vi "Drive Controller.vi"(8 "error in":errorcluster) -> ()   [LabVIEW 2017]
doc: "This VI executes continuously carrying out the current operation and responding to updates or new operation requests. It will often contain the timing or control code that is difficult to place directly in TeleOp. This VI generally opens all sensors and motors and isolates the rest of the robot code from knowing implementation details of how the operations are carried out."
uses:
  <vilib>/Rock Robotics/WPI/Framework/Completion Status.ctl
  Drive Setpoints.ctl
  Drive Operations.ctl
  Shared/RobotNeededPathData.ctl
  <vilib>/Rock Robotics/WPI/SafetyOutput/WPI_SafetyOutputConfigMenu.ctl
  <vilib>/Rock Robotics/SystemInterfaces/DIO/FPGA_DIOPWMChannel.ctl
  <vilib>/Rock Robotics/SystemInterfaces/DIO/FPGA_DIOChannel.ctl
  <vilib>/Rock Robotics/WPI/DriverStation/WPI_DriverStationRobotMode2.ctl
  <vilib>/Rock Robotics/WPI/ThirdParty/Sensors/navX/_TypeDefs/FRIC_navX_DeviceNumbersTypeDef.ctl
  <vilib>/Rock Robotics/WPI/RobotDrive/WPI_RobotDriveOpen4MotorWithSPARK.vi
  <vilib>/Rock Robotics/WPI/Counter/WPI_CounterDigitalInputToDigitalSource.vi
  <vilib>/Rock Robotics/WPI/RobotDrive/WPI_RobotDriveOpen2MotorWithSPARK.vi
  <vilib>/Rock Robotics/Network Tables/NT Write Number.vi
  Framework/Robot Global Data.vi
  Drive Published Globals.vi
  <vilib>/addons/control/pid/pid.llb/PID (DBL).vi
  <vilib>/addons/control/pid/NI_PID_pid.lvlib
  Configuration/Constants.vi
panel:
  in  "Integral Range":dbl=15.0
  out "PID Tuining":cluster{dbl, dbl}(graph)={170.0, 167.02}
  in  "Points":cluster{"X":dbl, "Y":dbl}[](array[cluster])=[{"X"=0.0, "Y"=0.0}, {"X"=0.01, "Y"=0.0}, {"X"=0.011, "Y"=0.17}, {"X"=1.0, "Y"=1.0}]
  in  "PID gains":T1={"proportional gain (Kc)"=0.01, "integral time (Ti, min)"=0.007, "derivative time (Td, min)"=0.0015} {"derivative time (Td, min)" format="%#_9g"}
  in  "Gains":T2={"FFV"=0.0059, "FFA"=0.0019, "Vel PID"={"P"=0.01, "I"=0.0, "D"=0.0}}
  in  "Interactive Values":T3={"Operation"=enum."Turn to Angle", "Left Speed"=-0.27, "Right Speed"=0.27, "Duration"=2.0, "Speed"=0.0, "Start Angle"=0.0, "Target Angle"=180.0, "Distance (inch)"=0.0, "Start Point (inch)"=0.0, "RobotNeededPathData"={"Path"=[], "MaxVel"=0.0, "MaxAccel"=-1.0, "Backwards?"=FALSE, "PointSpacing"=0.0, "LookaheadDist"=0.0, "Speed/Curve"=1.8, "SlowDistanceAtEnd"=12.0, "SlowSpeed"=15.0, "MaxDeAccel"=0.0}, "Start Point 2"=0.0} {"RobotNeededPathData"."SlowSpeed" format="%#_13g"; "RobotNeededPathData"."SlowDistanceAtEnd" format="%#_13g"; "RobotNeededPathData"."Speed/Curve" format="%#_13g"}
  in  "Buttons":cluster{"Execute Cmd":bool, "Abort Cmd":bool}
  out "Command Timing":cluster{"Start Time (ms)":u32, "Iterations":i32}={"Start Time (ms)"=372507, "Iterations"=0}
  out "Status":T6
  out "Setpoints":T7(graph)
  out "Current\nCmd":string="Started at  14:51:47.884\nDefault: Reserve,  L 0.0, R 0.0, D 0.000000"
  # "Tip: The graph shows the motor setpoints. It may also be helpful to observe inputs and sensor values.\nYou may also want to display tuning or debugging controls."
  # ".0088"
  # ".0017"
  # ".02"
  # "Interactive Command: You may fill in the settings for a command\nand schedule it with the Execute button. You can observe and abort\nany command while fine tuning the code for the controller."
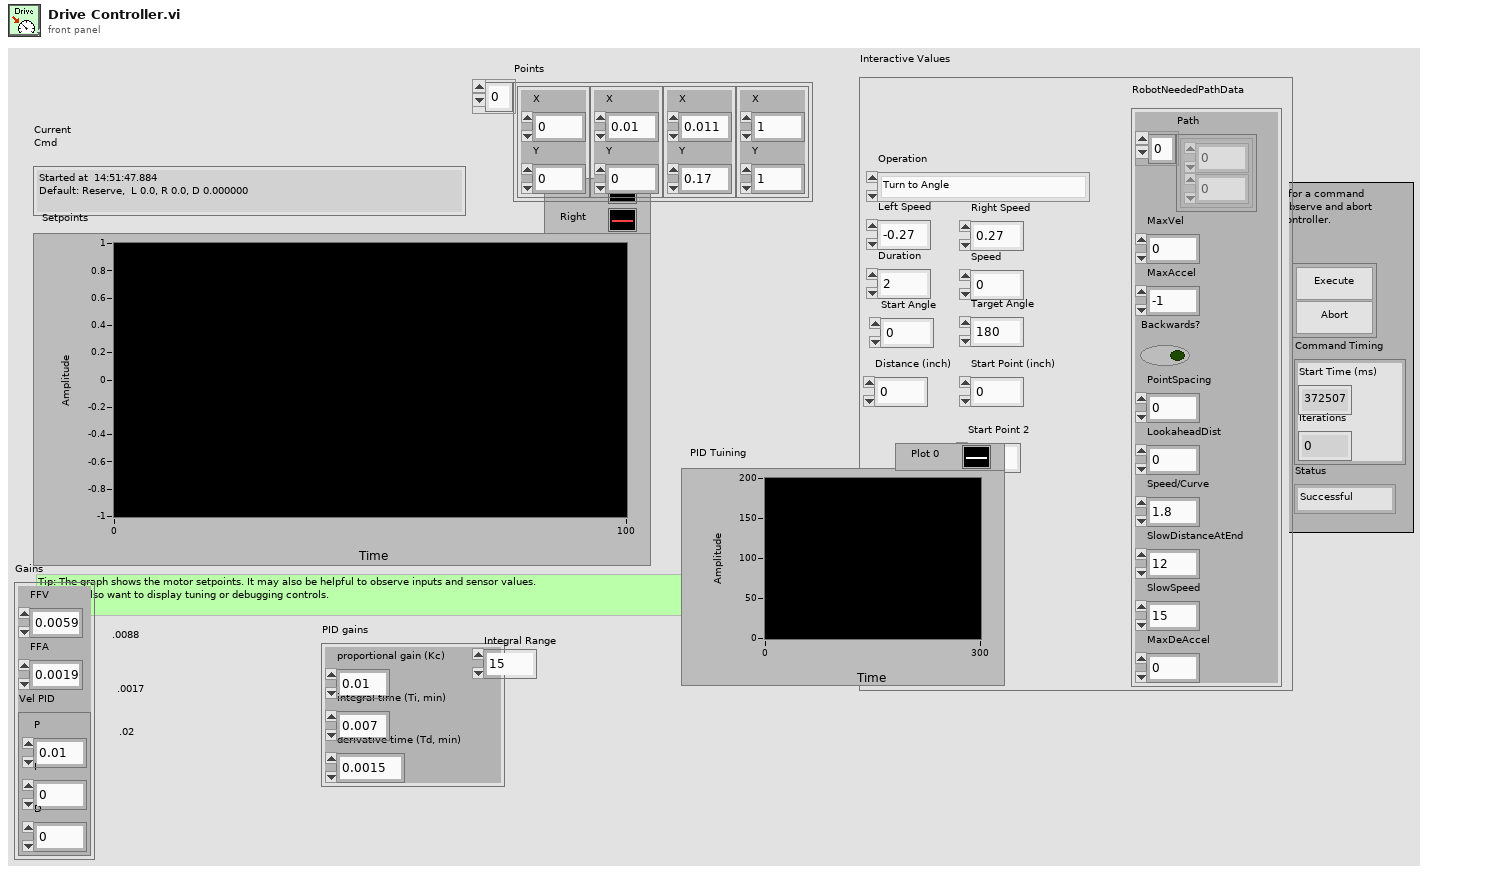
[diagram p1: front panel]
types:
  T1 = cluster{"proportional gain (Kc)":dbl, "integral time (Ti, min)":dbl, "derivative time (Td, min)":dbl}
  T2 = cluster{"FFV":dbl, "FFA":dbl, "Vel PID":cluster{"P":dbl, "I":dbl, "D":dbl}}
  T3 = typedef "Drive Setpoints.ctl" = cluster{"Operation":T4, "Left Speed":dbl, "Right Speed":dbl, "Duration":dbl, "Speed":dbl, "Start Angle":dbl, "Target Angle":dbl, "Distance (inch)":dbl, "Start Point (inch)":dbl, "RobotNeededPathData":T5, "Start Point 2":dbl}
  T4 = typedef "Drive Operations.ctl" = enum16{"Reserve", "Read Current", "Immediate", "Drive for Time", "Drive for Distance", "Turn to Angle", "Arc Turn", "Drive Path", "Drive To Cube"}
  T5 = typedef "RobotNeededPathData.ctl" = cluster{"Path":cluster{dbl, dbl}[], "MaxVel":dbl, "MaxAccel":dbl, "Backwards?":bool, "PointSpacing":dbl, "LookaheadDist":dbl, "Speed/Curve":dbl, "SlowDistanceAtEnd":dbl, "SlowSpeed":dbl, "MaxDeAccel":dbl}
  T6 = typedef "Completion Status.ctl" = enum16{"Successful", "Aborted", "Incomplete"}
  T7 = cluster{"Left Setpoint":dbl, "Right Setpoint":dbl}
  T8 = typedef "FPGA_DIOChannel.ctl" = enum8{"DIO 0", "DIO 1", "DIO 2", "DIO 3", "DIO 4", "DIO 5", "DIO 6", "DIO 7", "DIO 8", "DIO 9", "DIO MXP 0", "DIO MXP 1", "DIO MXP 2", "DIO MXP 3", "DIO MXP 4", "DIO MXP 5", "DIO MXP 6", "DIO MXP 7", "DIO MXP 8", "DIO MXP 9", "DIO MXP 10", "DIO MXP 11", "DIO MXP 12", "DIO MXP 13", "DIO MXP 14", "DIO MXP 15", "SPI Port CS1", "SPI Port CS2", "SPI Port CS3", "SPI Port MISO", "SPI Port MOSI", "Invalid"}
  T9 = typedef "FPGA_DIOPWMChannel.ctl" = enum8{"PWM 0", "PWM 1", "PWM 2", "PWM 3", "PWM 4", "PWM 5", "PWM 6", "PWM 7", "PWM 8", "PWM 9", "PWM MXP 0", "PWM MXP 1", "PWM MXP 2", "PWM MXP 3", "PWM MXP 4", "PWM MXP 5", "PWM MXP 6", "PWM MXP 7", "PWM MXP 8", "PWM MXP 9", "Invalid"}
  T10 = typedef "WPI_SafetyOutputConfigMenu.ctl" = enum16{"Enable", "Disable"}
  T11 = typedef "WPI_DigitalInputDevRef.ctl" = cluster{"DevStatus":errorcluster, "DIO Channel":T8}
  T12 = typedef "FPGA_CounterEncoderSourceConvertionLVSourceType.ctl" = cluster{"DevStatus":errorcluster, "AnalogTriggerMode?":bool, "DigitalMode":cluster{"DIO Channel":T13}, "AnalogTriggerMode":cluster{"AnalogTriggerIndex":T14, "OutputType":T15}}
  T13 = typedef "FPGA_DIODigitalSourceChannel.ctl" = enum8{"DIO 0", "DIO 1", "DIO 2", "DIO 3", "DIO 4", "DIO 5", "DIO 6", "DIO 7", "DIO 8", "DIO 9", "DIO MXP 0", "DIO MXP 1", "DIO MXP 2", "DIO MXP 3", "DIO MXP 4", "DIO MXP 5", "DIO MXP 6", "DIO MXP 7", "DIO MXP 8", "DIO MXP 9", "DIO MXP 10", "DIO MXP 11", "DIO MXP 12", "DIO MXP 13", "DIO MXP 14", "DIO MXP 15", "Disabled"}
  T14 = typedef "FPGA_AnalogTriggerIndex.ctl" = enum8{"Trig 0", "Trig 1", "Trig 2", "Trig 3", "Trig 4", "Trig 5", "Trig 6", "Trig 7", "Invalid"}
  T15 = typedef "FPGA_AnalogTriggerOutType.ctl" = enum16{"InWindow", "TriggerState", "Rising", "Falling"}
  T16 = typedef "WPI_RobotDriveDevRef.ctl" = cluster{"DevStatus":errorcluster, "Motors[]":T17[], "Square Inputs":bool, "Max Output":dbl}
  T17 = typedef "WPI_MotorControlDeviceRef.ctl" = cluster{"DeviceStatus":errorcluster, "Type":T18, "PWM":cluster{"PWM Channel":T9, "DeadBand":T19}, "CAN":cluster{"Device Number":u8, "SetOutput VI Ref":variant, "GetOutput VI Ref":variant, "Enable VI Ref":variant, "Disable VI Ref":variant, "Data":variant}, "Invert":bool, "DIO PWM":cluster{"PWM \"Enable\" Channel":T9, "DIOChannel":T8, "PWM Rate":dbl}}
  T18 = typedef "WPI_MotorControlType.ctl" = enum16{"PWM", "CAN", "DIO PWM"}
  T19 = typedef "WPI_PWMDeadband.ctl" = cluster{"Name":string, "maxPositivePwm":i32, "minPositivePwm":i32, "centerPwm":i32, "maxNegativePwm":i32, "minNegativePwm":i32, "angularRange":u16}
  T20 = typedef "WPI_EncoderDevRef.ctl" = cluster{"DevStatus":errorcluster, "EncoderIndex":T21, "CounterIndex":T22, "DistancePerCount":dbl, "Decoding Type":T23}
  T21 = typedef "FPGA_EncoderIdx.ctl" = enum8{"Enc 0", "Enc 1", "Enc 2", "Enc 3", "Enc 4", "Enc 5", "Enc 6", "Enc 7", "Invalid"}
  T22 = typedef "FPGA_CounterCtrSystemIndex.ctl" = enum8{"Ctr 0", "Ctr 1", "Ctr 2", "Ctr 3", "Ctr 4", "Ctr 5", "Ctr 6", "Ctr 7", "Invalid"}
  T23 = typedef "WPI_EncoderType.ctl" = enum16{"1x", "2x", "4x"}
  T24 = typedef "Command Status Info.ctl" = cluster{"Name":string, "Status":T6, "notifier out":T25}
  T25 = typedef "Completion Notifier.ctl" = refnum<notifier>
  T26 = cluster{"SubSystem Data":T3, cluster{"Start Time (ms)":u32, "Iterations":i32}, cluster{"Command Info":T24, "Description":string, "Default Command":T3, "queue out":refnum<queue>, "Subsystem Name":string}}
  T27 = typedef "WPI_DriverStationRobotMode2.ctl" = enum16{"Autonomous Disabled", "Autonomous Enabled", "Teleop Disabled", "Teleop Enabled", "Disconnected", "Finish", "Test Disabled", "Test Enabled", "Emergency Stopped"}
  T28 = cluster{"Yaw":dbl, "Roll":dbl, "Pitch":dbl, "Heading":dbl, "Fused Heading":dbl}
  T29 = typedef "FRIC_navX_DeviceNumbersTypeDef.ctl" = enum16{"Dev0", "Dev1", "Dev2", "Dev3"}
  T30 = cluster{"dx/dt":dbl, "dx/dt":dbl, "Yaw":dbl, cluster{dbl, dbl}}
  T31 = cluster{"LeftDistance":dbl, "RightDistance":dbl, "LeftVelocity":dbl, "RightVelocity":dbl, "Angle":dbl, "Location":cluster{dbl, dbl}}
  T32 = cluster{"SubSystem Data":T3, cluster{"Start Time (ms)":u32, "Iterations":i32}, "Default Command Arguments":cluster{"Command Info":T24, "Description":string, "Default Command":T3, "queue out":refnum<queue>, "Subsystem Name":string}}
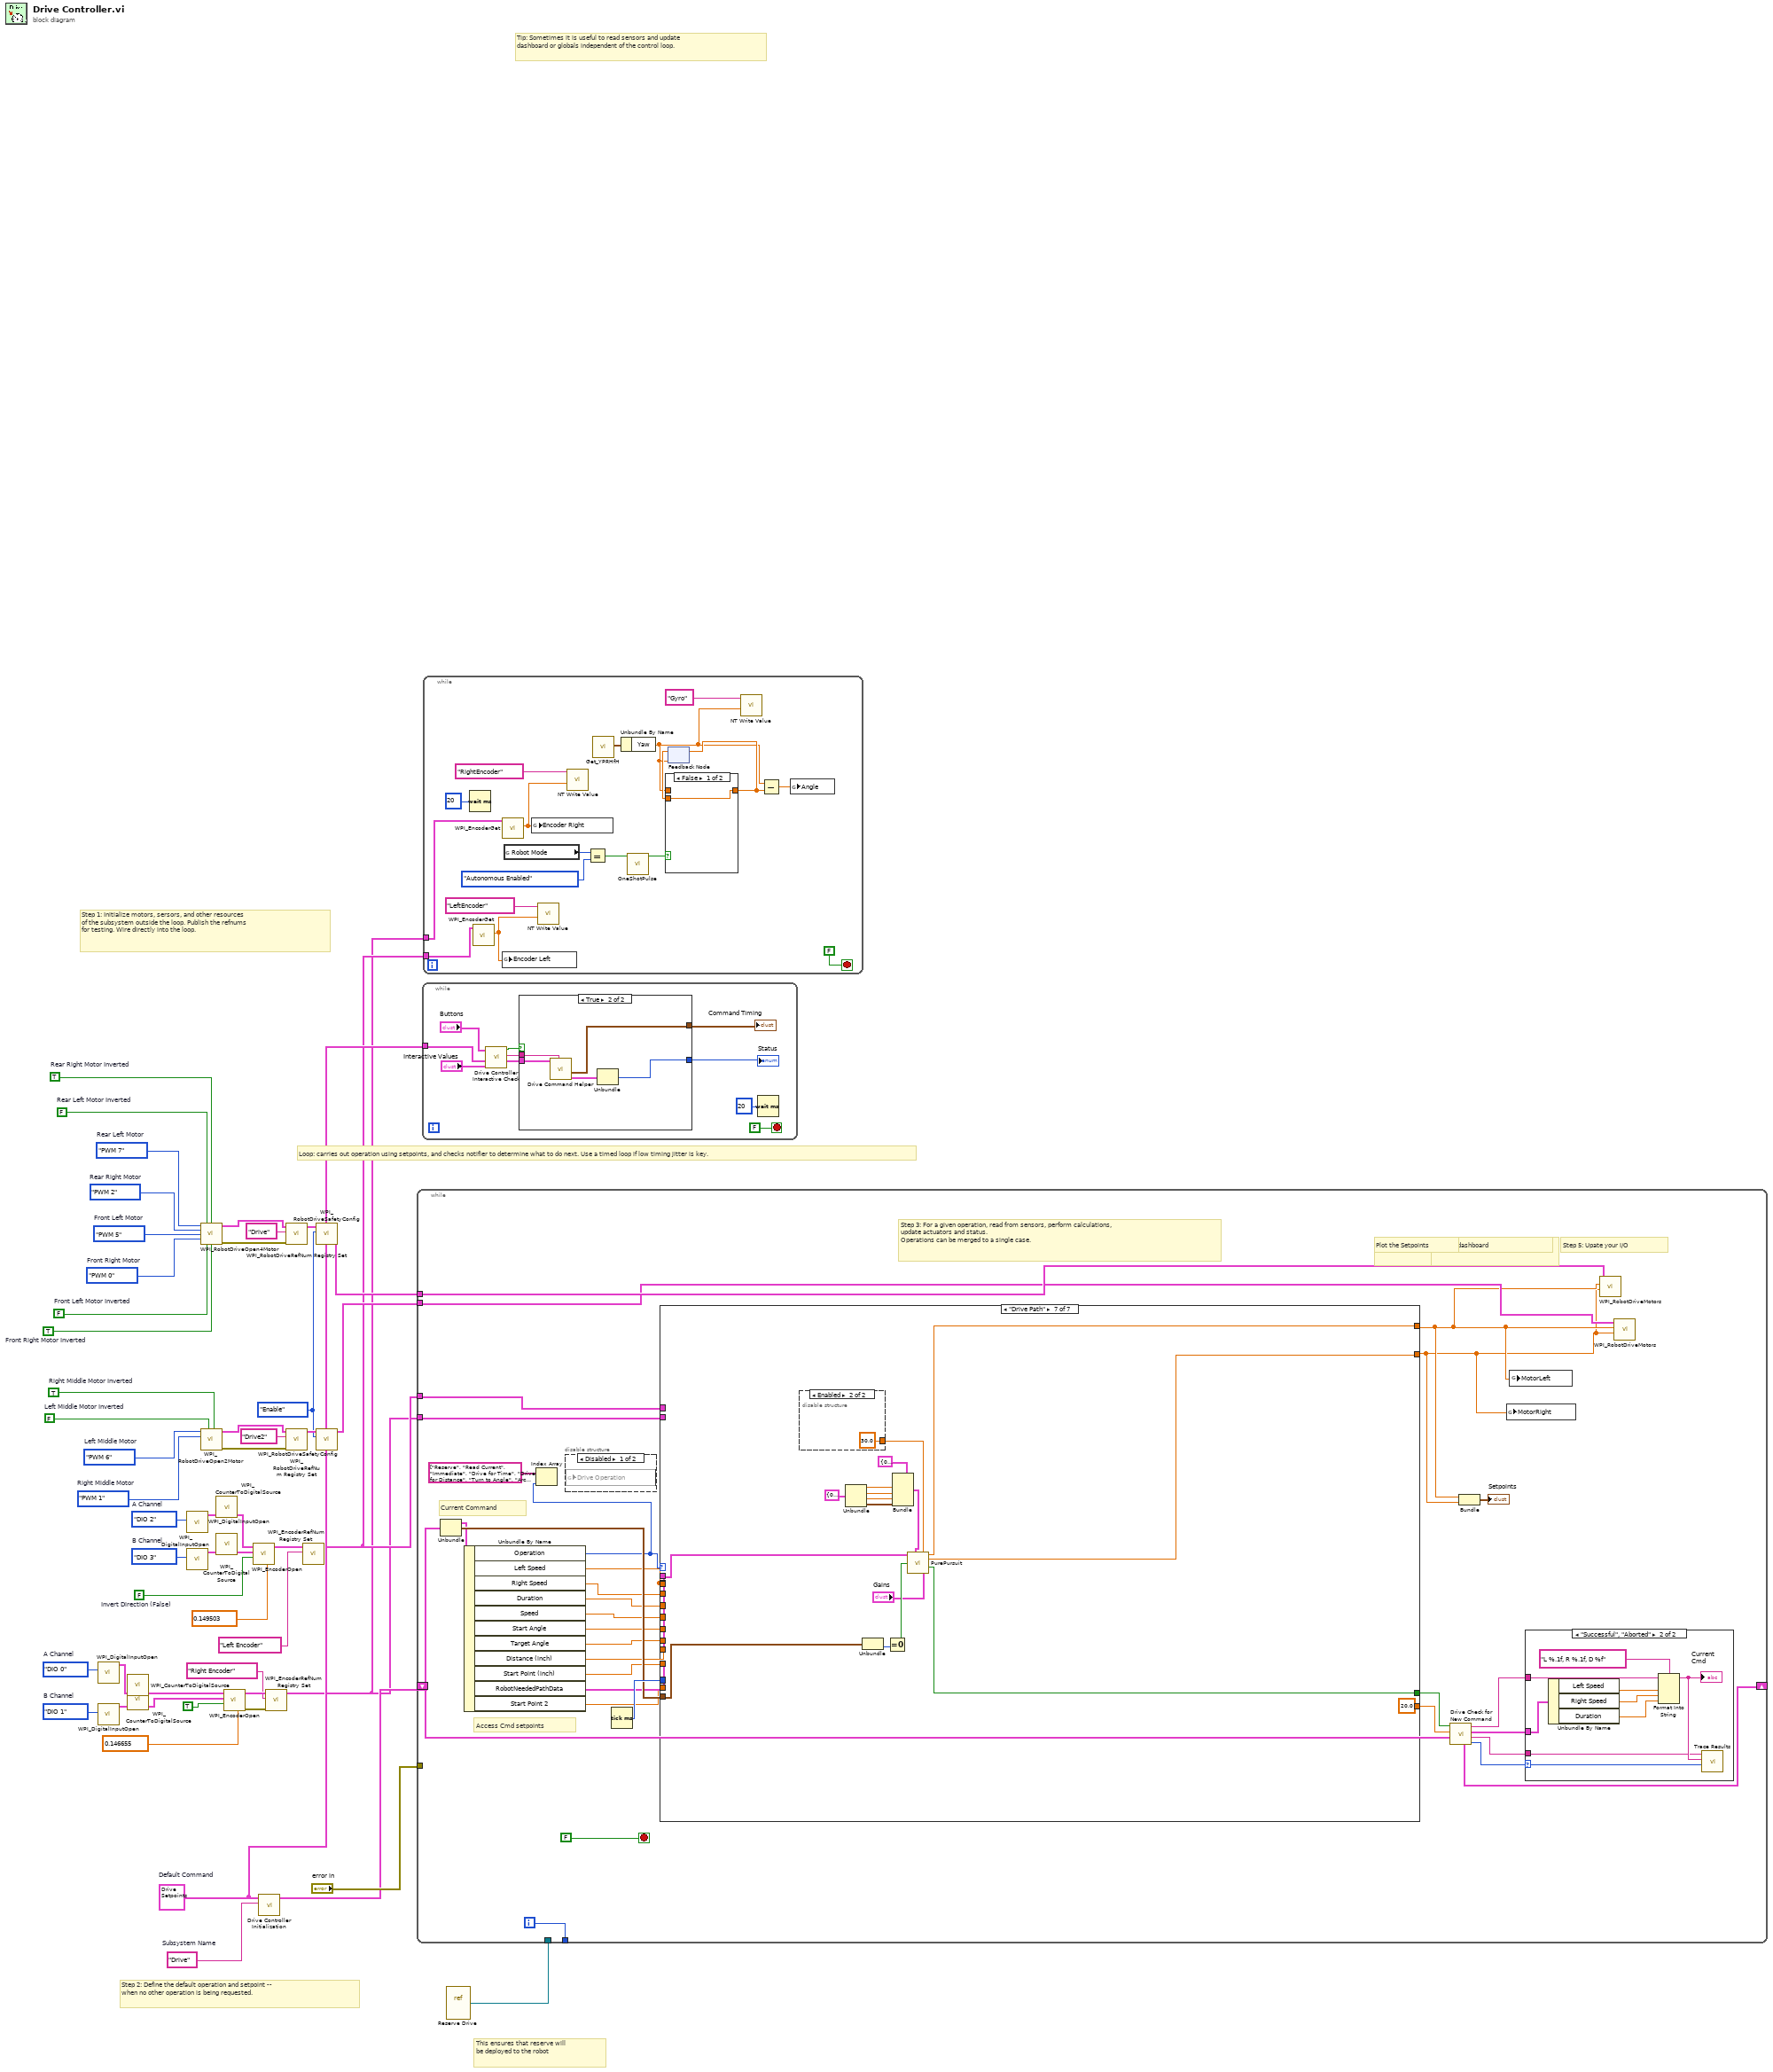
[diagram p0: block diagram]
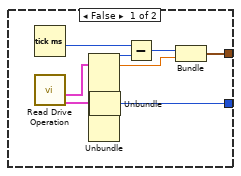
[diagram p3: hidden frame]
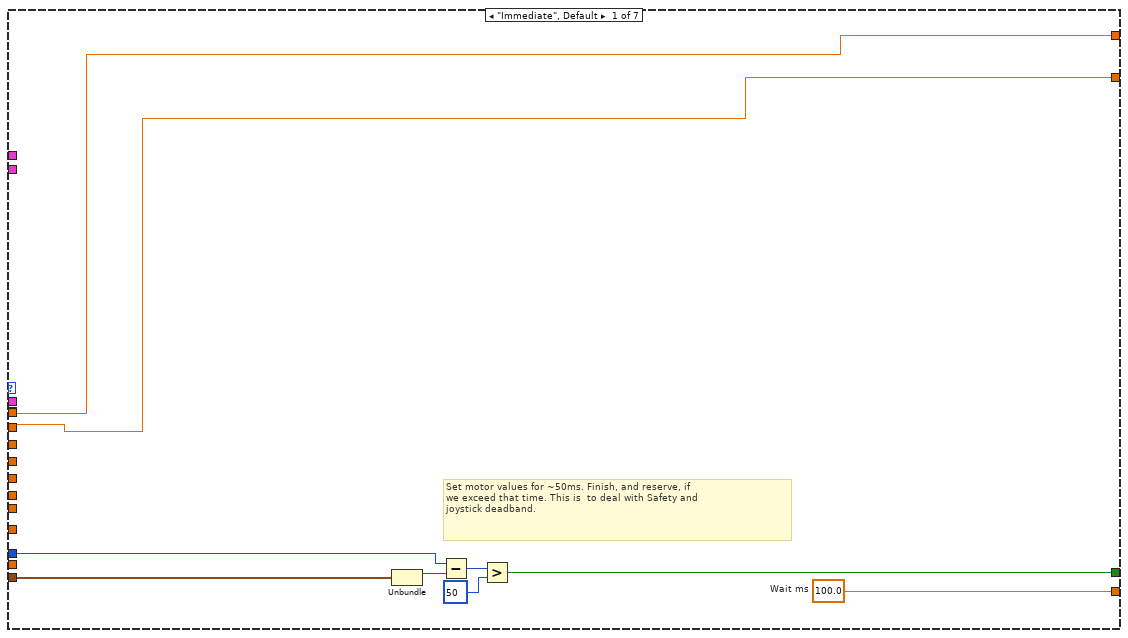
[diagram p5: hidden frame]
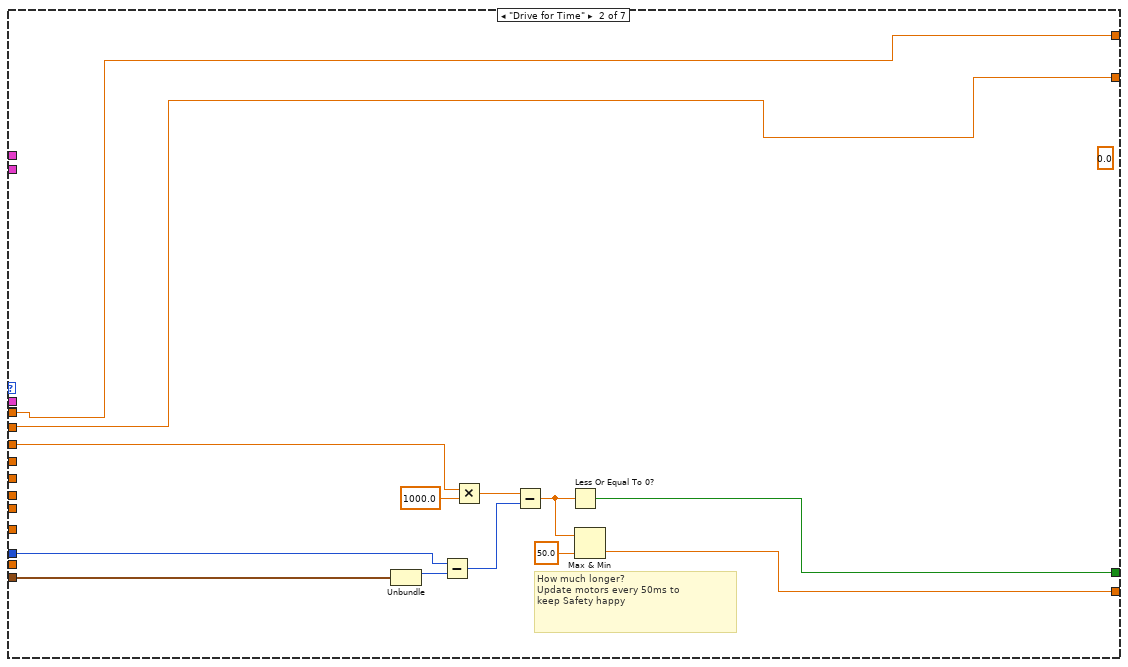
[diagram p6: hidden frame]
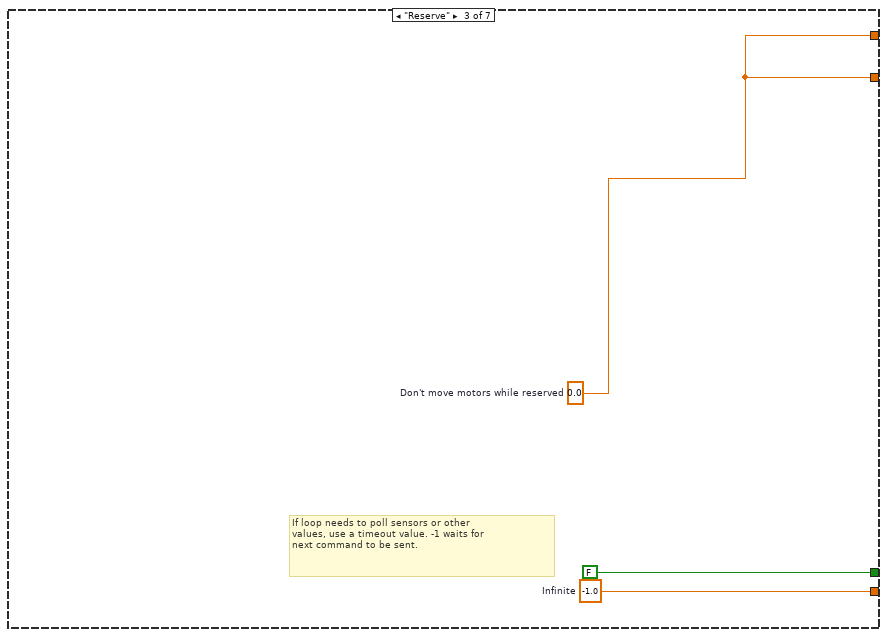
[diagram p7: hidden frame]
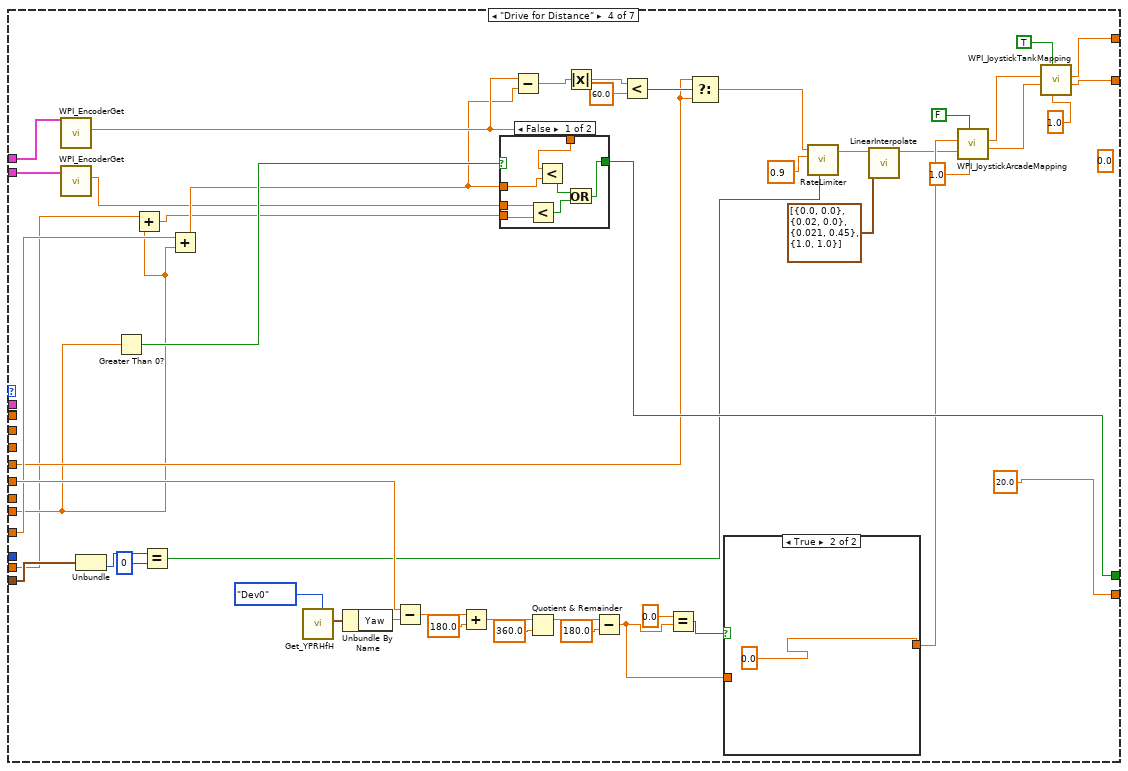
[diagram p8: hidden frame]
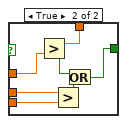
[diagram p9: hidden frame]
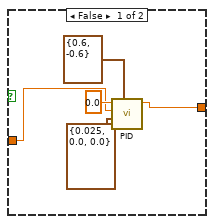
[diagram p10: hidden frame]
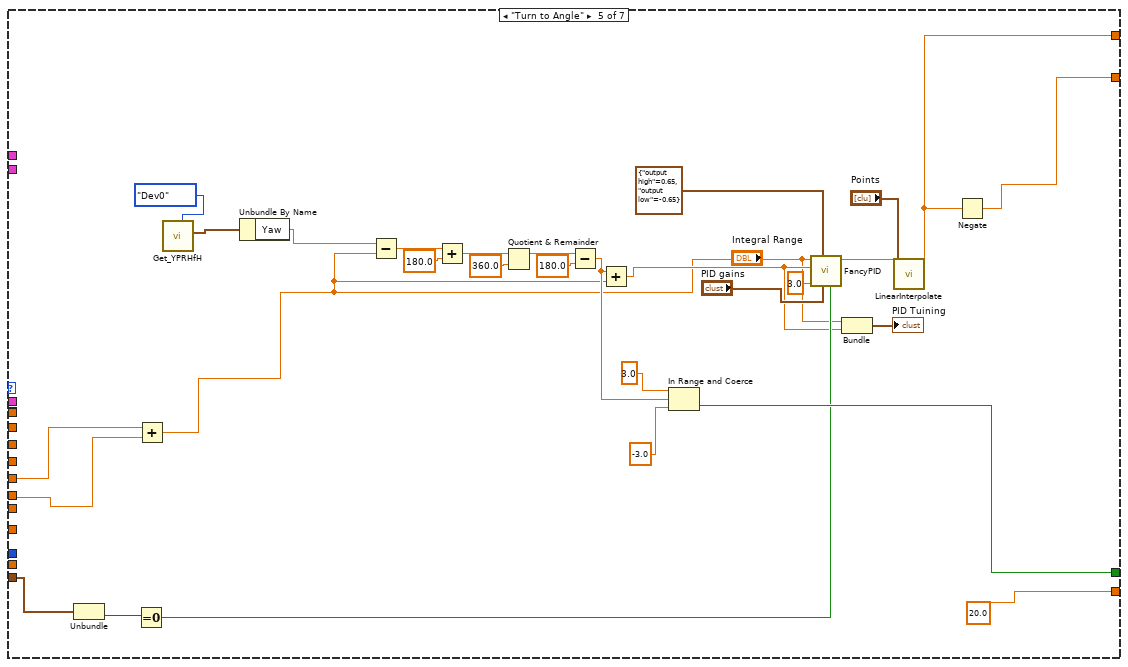
[diagram p11: hidden frame]
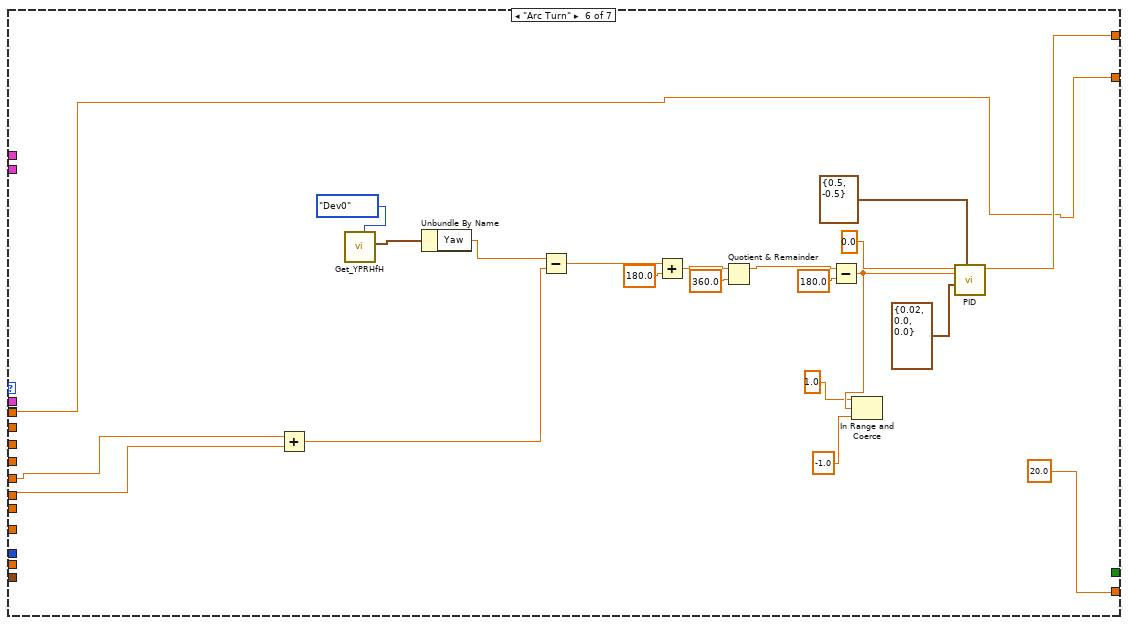
[diagram p12: hidden frame]
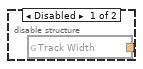
[diagram p13: hidden frame]
diagram:
  w6 = FPGA_DIOChannel."DIO 1"  # B Channel
  w9 = FPGA_DIOChannel."DIO 0"  # A Channel
  w14 = T3 {"Operation"=enum."Reserve", "Left Speed"=0.0, "Right Speed"=0.0, "Duration"=0.0, "Speed"=0.0, "Start Angle"=0.0, "Target Angle"=0.0, "Distance (inch)"=0.0, "Start Point (inch)"=0.0, "RobotNeededPathData"={"Path"=[], "MaxVel"=0.0, "MaxAccel"=0.0, "Backwards?"=FALSE, "PointSpacing"=0.0, "LookaheadDist"=0.0, "Speed/Curve"=1.8, "SlowDistanceAtEnd"=12.0, "SlowSpeed"=15.0, "MaxDeAccel"=0.0}, "Start Point 2"=0.0}  # Default Command
  w21 = TRUE  # Right Middle Motor Inverted
  w22 = FALSE  # Left Middle Motor Inverted
  w25 = FPGA_DIOPWMChannel."PWM 1"  # Right Middle Motor
  w26 = FPGA_DIOPWMChannel."PWM 6"  # Left Middle Motor
  w34 = FALSE  # Invert Direction (False)
  w27 = FPGA_DIOChannel."DIO 3"  # B Channel
  w28 = FPGA_DIOChannel."DIO 2"  # A Channel
  w36 = TRUE  # Front Right Motor Inverted
  w37 = FALSE  # Front Left Motor Inverted
  w38 = TRUE  # Rear Right Motor Inverted
  w39 = FALSE  # Rear Left Motor Inverted
  w40 = FPGA_DIOPWMChannel."PWM 0"  # Front Right Motor
  w41 = FPGA_DIOPWMChannel."PWM 5"  # Front Left Motor
  w42 = FPGA_DIOPWMChannel."PWM 2"  # Rear Right Motor
  w43 = FPGA_DIOPWMChannel."PWM 7"  # Rear Left Motor
  w16 = WPI_SafetyOutputConfigMenu."Enable" ("mode")
  w51 = "Drive"  # Subsystem Name
  # "Step 1: Initialize motors, sersors, and other resources\nof the subsystem outside the loop. Publish the refnums\nfor testing. Wire directly into the loop."
  # "Step 2: Define the default operation and setpoint --\nwhen no other operation is being requested."
  # "This ensures that reserve will\nbe deployed to the robot"
  # "Tip: Sometimes it is useful to read sensors and update\ndashboard or globals independent of the control loop."
  # "Loop: carries out operation using setpoints, and checks notifier to determine what to do next. Use a timed loop if low timing jitter is key."
  n1 = call <vilib>:"WPI_DigitalInputOpen.vi"("DIO Channel"=w9) -> ("DigitalInputDevRef"=w10:T11)  [unwired: 1 in, 9 out]
  n2 = call <vilib>:"WPI_DigitalInputOpen.vi"("DIO Channel"=w6) -> ("DigitalInputDevRef"=w7:T11)  [unwired: 1 in, 9 out]
  n3 = call-poly <vilib>:"WPI_CounterToDigitalSource.vi"("DigitalInputDevRef"=w10) -> ("Digital Source"=w11:T12)  [unwired: 6 out]
  n4 = call-poly <vilib>:"WPI_CounterToDigitalSource.vi"("DigitalInputDevRef"=w7) -> ("Digital Source"=w8:T12)  [unwired: 6 out]
  n5 = call <vilib>:"WPI_DigitalInputOpen.vi"("DIO Channel"=w28) -> ("DigitalInputDevRef"=w31:T11)  [unwired: 1 in, 9 out]
  n6 = call <vilib>:"WPI_DigitalInputOpen.vi"("DIO Channel"=w27) -> ("DigitalInputDevRef"=w30:T11)  [unwired: 1 in, 9 out]
  n7 = call-poly <vilib>:"WPI_RobotDriveOpen4Motor.vi"("Rear Left Motor"=w43, "Rear Left Motor Inverted"=w39, "Rear Right Motor Inverted"=w38, "Rear Right Motor"=w42, "Front Left Motor"=w41, "Front Right Motor"=w40, "Front Left Motor Inverted"=w37, "Front Right Motor Inverted"=w36) -> ("RobotDriveDevRef"=w50:T16, "error out"=w48:errorcluster)  [unwired: 6 in]
  n8 = call-poly <vilib>:"WPI_RobotDriveOpen2Motor.vi"("Right Motor Inverted"=w21, "Left Motor Inverted"=w22, "Right Motor"=w25, "Left Motor"=w26) -> ("error out"=w20:errorcluster, "RobotDriveDevRef"=w24:T16)  [unwired: 6 in]
  n9 = call-poly <vilib>:"WPI_CounterToDigitalSource.vi"("DigitalInputDevRef"=w31) -> ("Digital Source"=w32:T12)  [unwired: 6 out]
  n10 = call-poly <vilib>:"WPI_CounterToDigitalSource.vi"("DigitalInputDevRef"=w30) -> ("Digital Source"=w29:T12)  [unwired: 6 out]
  n11 = call <vilib>:"WPI_EncoderOpen.vi"("DistancePerCount"=0.146655, "Invert Direction (False)"=TRUE, "BSource"=w8, "ASource"=w11) -> ("error out"=w13:errorcluster, "EncoderDevRef"=w12:T20)  [unwired: 4 in, 2 out]
  n12 = call <vilib>:"WPI_EncoderOpen.vi"("DistancePerCount"=0.149503, "Invert Direction (False)"=w34, "BSource"=w29, "ASource"=w32) -> ("EncoderDevRef"=w33:T20)  [unwired: 4 in, 3 out]
  n13 = call "Drive Controller Initialization.vi"("Subsystem Name"=w51, "Default Command"=w14) -> ("Current Command"=w45:T26)  [unwired: 9 in]
  n14 = call <vilib>:"WPI_EncoderRefNum Registry Set.vi"("error in (no error)"=w13, "refnum name"="Right Encoder", "EncoderDevRef"=w12) -> ("EncoderDevRef"=w1:T20)  [unwired: 7 in, 1 out]
  n15 = call <vilib>:"WPI_RobotDriveRefNum Registry Set.vi"("error in (no error)"=w48, "refnum name"="Drive", "RobotDriveDevRef"=w50) -> ("RobotDriveDevRef"=w19:T16)  [unwired: 1 in, 7 out]
  n16 = call <vilib>:"WPI_RobotDriveRefNum Registry Set.vi"("error in (no error)"=w20, "refnum name"="Drive2", "RobotDriveDevRef"=w24) -> ("RobotDriveDevRef"=w18:T16)  [unwired: 7 in, 1 out]
  n17 = call <vilib>:"WPI_EncoderRefNum Registry Set.vi"("refnum name"="Left Encoder", "EncoderDevRef"=w33) -> ("EncoderDevRef"=w2:T20)  [unwired: 8 in, 1 out]
  n18 = call <vilib>:"WPI_RobotDriveSafetyConfig.vi"("mode"=w16, "RobotDriveDevRef"=w19) -> ("RobotDriveDevRef"=w47:T16)  [unwired: 8 in, 1 out]
  n19 = call <vilib>:"WPI_RobotDriveSafetyConfig.vi"("mode"=w16, "RobotDriveDevRef"=w18) -> ("RobotDriveDevRef"=w17:T16)  [unwired: 8 in, 1 out]
  n20 = while {
    tunnel: w14 -> [w53]
    stop <- FALSE stop-if-true
    n21 = call "Drive Controller Interactive Check.vi"("Interactive Command In"="Interactive Values", "Default Command"=w53, "Buttons"="Buttons") -> ("Interactive Command Out"=w55:T3, "Trace String"=w56:string, "Schedule"=w57:bool)  [unwired: 6 in]
    n22 = case shown="True" w57 {
      tunnel: [w66 w74] -> w58
      tunnel: [w65 w70] -> w59
      tunnel: w56 -> [_ w72]
      tunnel: w55 -> [_ w71]
      frame False {
        n23 = Tick Count (ms)() -> (millisecond timer value=w69:u32)
        n24 = call "Read Drive Operation.vi"() -> ("Command Info"=w63:T24, "SubSystem Data"=w62:T3)  [unwired: 9 in, 1 out]
        n25 = Unbundle(w62) -> ("Operation"=w67:T4, "Left Speed"=w64:dbl)  [unwired: 9 out]
        n26 = Unbundle(w63) -> ("Status"=w66:T6)  [unwired: 2 out]
        n27 = Subtract(x=w69, y=w67) -> (x-y=w68:u32)
        n28 = Bundle(w68, "Left Speed"=w64) -> (w65:cluster{u32, "Left Speed":dbl})  [unwired: 1 in]
      }
      frame True {
        n29 = call "Drive Command Helper.vi"("Description"=w72, "SubSystem Data"=w71) -> ("Command Info Out"=w73:T24, "Command Timing"=w70:cluster{"Start Time (ms)":u32, "Iterations":i32})  [unwired: 7 in, 1 out]
        n30 = Unbundle(w73) -> ("Status"=w74:T6)  [unwired: 2 out]
      }
    }
    "Status" <- w58
    "Command Timing" <- w59
    n31 = Wait (ms)(milliseconds to wait=u32 20) -> ()  [unwired: 1 out]
  }
  n32 = while {
    tunnel: w2 -> [w76]
    tunnel: w1 -> [w75]
    stop <- FALSE stop-if-true
    n33 = Wait (ms)(milliseconds to wait=u32 20) -> ()  [unwired: 1 out]
    n34 = call <vilib>:"WPI_EncoderGet.vi"("EncoderDevRef"=w76) -> ("Distance"=w82:dbl)  [unwired: 5 in, 5 out]
    n35 = call <vilib>:"WPI_EncoderGet.vi"("EncoderDevRef"=w75) -> ("Distance"=w80:dbl)  [unwired: 5 in, 5 out]
    n36 = global write "Drive Published Globals.vi" "Encoder Left"(w82) -> ()
    n37 = global read "Robot Global Data.vi" "Robot Mode"() -> (w87:T27)
    n38 = global write "Drive Published Globals.vi" "Encoder Right"(w80) -> ()
    n39 = call-poly <vilib>:"NT Write Value.vi"("Numeric"=w82, "Name"="LeftEncoder") -> ()  [unwired: 9 in, 1 out]
    n40 = call-poly <vilib>:"NT Write Value.vi"("Numeric"=w80, "Name"="RightEncoder") -> ()  [unwired: 9 in, 1 out]
    n41 = Equal?(x=w87, y=WPI_DriverStationRobotMode2."Autonomous Enabled") -> (x = y?=w78:bool)
    n42 = call <vilib>:"Get_YPRHfH.vi"() -> ("YRPHfH"=w92:T28)  [unwired: 11 in]
    n43 = Unbundle By Name(w92) -> ("Yaw"=w79:dbl)
    n44 = call "OneShotPulse.vi"("Input"=w78) -> ("Output"=w77:bool)  [unwired: 10 in]
    n45 = feedback #1(w79) -> (w88:dbl)
    n46 = case shown="False" w77 {
      tunnel: w79 -> [_ w94]
      tunnel: [w93 w94] -> w89
      tunnel: w88 -> [w93 _]
      frame False {
      }
      frame True {
      }
    }
    n47 = feedback-in #1(w89) -> ()
    n48 = call-poly <vilib>:"NT Write Value.vi"("Numeric"=w79, "Name"="Gyro") -> ()  [unwired: 9 in, 1 out]
    n49 = Subtract(x=w79, y=w89) -> (x-y=w84:dbl)
    n50 = global write "Drive Published Globals.vi" "Angle"(w84) -> ()
  }
  n51 = vi-ref "Reserve Drive.vi"() -> (w44:refnum<vi>)
  n52 = while {
    shift-right: [w122] -> _
    shift-left: w45 -> [w95]
    tunnel: [w125] -> _
    tunnel: w47 -> [w104]
    tunnel: "error in" -> [_]
    tunnel: w44 -> [_]
    tunnel: w2 -> [w102]
    tunnel: w17 -> [w103]
    tunnel: w1 -> [w101]
    i -> [w125]
    stop <- FALSE stop-if-true
    # "Plot the Setpoints"
    # "Step 5: Upate your I/O"
    # "Step 4: Format a string to describe this\ncmd and how the previous cmd finished"
    # "Current Command"
    # "Update motors and update dashboard"
    # "Access Cmd setpoints"
    # "Finished? &\nWait Time"
    # "Step 3: For a given operation, read from sensors, perform calculations,\nupdate actuators and status.\nOperations can be merged to a single case."
    n53 = Unbundle(w95) -> ("SubSystem Data"=w105:T3, w116:cluster{"Start Time (ms)":u32, "Iterations":i32})  [unwired: 1 out]
    n54 = Unbundle By Name(w105) -> ("Operation"=w97:T4, "Left Speed"=w114:dbl, "Right Speed"=w113:dbl, "Duration"=w112:dbl, "Speed"=w111:dbl, "Start Angle"=w110:dbl, "Target Angle"=w109:dbl, "Distance (inch)"=w108:dbl, "Start Point (inch)"=w107:dbl, "RobotNeededPathData"=w106:T5, "Start Point 2"=w100:dbl)
    n55 = Index Array(array=string[] ["Reserve", "Read Current", "Immediate", "Drive for Time", "Drive for Distance", "Turn to Angle", "Arc Turn", "Drive Path", "Drive To Cube"] ("Strings []"), index=w97) -> ()  [unwired: 1 out]
    n56 = disable-structure shown="Disabled" {
      frame Disabled {
        n57 = global read "Robot Global Data.vi" "Drive Operation"() -> ()  [unwired: 1 in]
      }
      frame Enabled {
      }
    }
    n58 = Tick Count (ms)() -> (millisecond timer value=w124:u32)
    n59 = case shown="\"Drive Path\"" w97 {
      tunnel: [w135 w139 w151 20.0 ("Infinite") 20.0 ("Infinite") 20.0 ("Infinite") 20.0 ("Infinite")] -> w121
      tunnel: [w130 w143 FALSE ("ignore previous (F)") w187 w242 _ w284] -> w120
      tunnel: w116 -> [w129 w145 _ w168 w232 _ w283]
      tunnel: w124 -> [w131 w142 _ _ _ _ _]
      tunnel: [w128 w137 w149 w173 w230 w251 w286] -> w99
      tunnel: [w127 w136 w149 w174 w229 w250 w285] -> w98
      tunnel: w111 -> [_ _ _ w157 _ _ _]
      tunnel: w108 -> [_ _ _ w155 _ _ _]
      tunnel: w112 -> [_ w138 _ _ _ _ _]
      tunnel: w114 -> [w128 _ _ _ _ w250 _]
      tunnel: w113 -> [w127 w136 _ _ _ _ _]
      tunnel: w102 -> [_ _ _ w185 _ _ _]
      tunnel: w110 -> [_ _ _ w181 w245 w254 _]
      tunnel: w109 -> [_ _ _ _ w244 w253 _]
      tunnel: w107 -> [_ _ _ w180 _ _ _]
      tunnel: w114 -> [_ w137 _ _ _ _ _]
      tunnel: w106 -> [_ _ _ _ _ _ w287]
      tunnel: w101 -> [_ _ _ w156 _ _ _]
      tunnel: w100 -> [_ _ _ w154 _ _ _]
      frame "Immediate", Default {
        w135 = 100.0  # Wait ms
        # "Set motor values for ~50ms. Finish, and reserve, if\nwe exceed that time. This is  to deal with Safety and\njoystick deadband."
        n60 = Unbundle(w129) -> ("Start Time (ms)"=w132:u32)  [unwired: 1 out]
        n61 = Subtract(x=w131, y=w132) -> (x-y=w133:u32)
        n62 = Greater?(x=w133, y=u8 50 ("Left Motor")) -> (0:w130:bool)
      }
      frame "Drive for Time" {
        (unwired) 0.0 ("output")
        # "How much longer?\nUpdate motors every 50ms to\nkeep Safety happy"
        n63 = Unbundle(w145) -> ("Start Time (ms)"=w144:u32)  [unwired: 1 out]
        n64 = Subtract(x=w142, y=w144) -> (x-y=w148:u32)
        n65 = Multiply(x=w138, y=1000.0) -> (x*y=w147:dbl)
        n66 = Subtract(x=w147, y=w148) -> (x-y=w141:dbl)
        n67 = Less Or Equal To 0?(x=w141) -> (x <= 0?=w143:bool)
        n68 = Max & Min(x=w141, y=50.0) -> (min(x,y)=w139:dbl)  [unwired: 1 out]
      }
      frame "Reserve" {
        w149 = 0.0  # Don't move motors while reserved
        w151 = -1.0  # Infinite
        # "If loop needs to poll sensors or other\nvalues, use a timeout value. -1 waits for\nnext command to be sent."
      }
      frame "Drive for Distance" {
        (unwired) 0.0 ("output")
        n69 = call <vilib>:"WPI_EncoderGet.vi"("EncoderDevRef"=w185) -> ("Distance"=w164:dbl)  [unwired: 5 in, 5 out]
        n70 = call <vilib>:"WPI_EncoderGet.vi"("EncoderDevRef"=w156) -> ("Distance"=w152:dbl)  [unwired: 5 in, 5 out]
        n71 = Unbundle(w168) -> ("Iterations"=w167:i32)  [unwired: 1 out]
        n72 = Greater Than 0?(x=w155) -> (x > 0?=w179:bool)
        n73 = Add(x=w154, y=w155) -> (x+y=w153:dbl)
        n74 = Equal?(x=w167, y=0) -> (x = y?=w165:bool)
        n75 = Add(x=w180, y=w155) -> (x+y=w163:dbl)
        n76 = call <vilib>:"Get_YPRHfH.vi"("Device Number"=FRIC_navX_DeviceNumbersTypeDef."Dev0") -> ("YRPHfH"=w199:T28)  [unwired: 10 in]
        n77 = Unbundle By Name(w199) -> ("Yaw"=w190:dbl)
        n78 = Subtract(x=w181, y=w190) -> (x-y=w189:dbl)
        n79 = Add(x=w189, y=180.0) -> (x+y=w194:dbl)
        n80 = case shown="False" w179 {
          tunnel: w164 -> [w205 w213]
          tunnel: w163 -> [w206 w212]
          tunnel: [w203 w207] -> w187
          tunnel: w153 -> [w201 w211]
          tunnel: w152 -> [w202 w210]
          frame False {
            n81 = Less?(x=w202, y=w201) -> (x < y?=w200:bool)
            n82 = Less?(x=w205, y=w206) -> (x < y?=w204:bool)
            n83 = Or(x=w204, y=w200) -> (x .or. y?=w203:bool)
          }
          frame True {
            n84 = Greater?(x=w213, y=w212) -> (0:w209:bool)
            n85 = Greater?(x=w210, y=w211) -> (0:w208:bool)
            n86 = Or(x=w209, y=w208) -> (x .or. y?=w207:bool)
          }
        }
        n87 = Subtract(x=w164, y=w163) -> (x-y=w162:dbl)
        n88 = Quotient & Remainder(x=w194, y=360.0) -> (x-y*floor(x/y)=w192:dbl)  [unwired: 1 out]
        n89 = Absolute Value(x=w162) -> (abs(x)=w161:dbl)
        n90 = Subtract(x=w192, y=180.0) -> (x-y=w188:dbl)
        n91 = Less?(x=w161, y=60.0) -> (x < y?=w159:bool)
        n92 = Equal?(x=0.0, y=w188) -> (x = y?=w197:bool)
        n93 = Select(t=w157, s=w159, f=w157) -> (s? t:f=w158:dbl)
        n94 = case shown="True" w197 {
          tunnel: [w214 0.0] -> w182
          tunnel: w188 -> [w215 _]
          frame False {
            n95 = call-poly <vilib>:"PID.vi"("output range"=cluster{"output high":dbl, "output low":dbl} {"output high"=0.6, "output low"=-0.6}, "PID gains"=T1 {"proportional gain (Kc)"=0.025, "integral time (Ti, min)"=0.0, "derivative time (Td, min)"=0.0}, "process variable"=w215, "setpoint"=0.0) -> ("output"=w214:dbl)  [unwired: 6 in, 1 out]
          }
          frame True {
          }
        }
        n96 = call "RateLimiter.vi"("Reset"=w165, "Max dx/dt"=0.9, "Input"=w158) -> ("Output"=w176:dbl)  [unwired: 8 in]
        n97 = call "LinearInterpolate.vi"("Points"=cluster{"X":dbl, "Y":dbl}[] [{"X"=0.0, "Y"=0.0}, {"X"=0.02, "Y"=0.0}, {"X"=0.021, "Y"=0.45}, {"X"=1.0, "Y"=1.0}], "Value"=w176) -> ("Output"=w177:dbl)  [unwired: 9 in]
        n98 = call <vilib>:"WPI_JoystickArcadeMapping.vi"("Max Output"=1.0, "Square Inputs"=FALSE, "Y axis value"=w177, "X axis value"=w182) -> ("Right Motor Value"=w172:dbl, "Left Motor Value"=w171:dbl)  [unwired: 6 in]
        n99 = call <vilib>:"WPI_JoystickTankMapping.vi"("Max Output"=1.0, "Square Inputs"=TRUE, "Right axis value"=w172, "Left axis value"=w171) -> ("Right Motor Value"=w174:dbl, "Left Motor Value"=w173:dbl)  [unwired: 6 in]
      }
      frame "Turn to Angle" {
        n100 = Unbundle(w232) -> ("Iterations"=w231:i32)  [unwired: 1 out]
        n101 = Equal To 0?(x=w231) -> (x = 0?=w225:bool)
        n102 = Add(x=w245, y=w244) -> (x+y=w222:dbl)
        n103 = call <vilib>:"Get_YPRHfH.vi"("Device Number"=FRIC_navX_DeviceNumbersTypeDef."Dev0") -> ("YRPHfH"=w247:T28)  [unwired: 10 in]
        n104 = Unbundle By Name(w247) -> ("Yaw"=w235:dbl)
        n105 = Subtract(x=w235, y=w222) -> (x-y=w236:dbl)
        n106 = Add(x=w236, y=180.0) -> (x+y=w239:dbl)
        n107 = Quotient & Remainder(x=w239, y=360.0) -> (x-y*floor(x/y)=w237:dbl)  [unwired: 1 out]
        n108 = Subtract(x=w237, y=180.0) -> (x-y=w234:dbl)
        n109 = Add(x=w234, y=w222) -> (x+y=w223:dbl)
        n110 = In Range and Coerce(upper limit=3.0, x=w234, lower limit=-3.0) -> (In Range?=w242:bool)  [unwired: 1 out]
        n111 = call "FancyPID.vi"("Reset"=w225, "Gains"="PID gains", "Range"=cluster{"output high":dbl, "output low":dbl} {"output high"=0.65, "output low"=-0.65} ("output range"), "Disable Range"=3.0, "Integral Range"="Integral Range", "Process variable"=w223, "Setpoint"=w222) -> ("output"=w226:dbl)  [unwired: 4 in]
        n112 = Bundle(w222, w223) -> (→"PID Tuining":cluster{dbl, dbl})  [unwired: 1 in]
        n113 = call "LinearInterpolate.vi"("Points"="Points", "Value"=w226) -> ("Output"=w230:dbl)  [unwired: 9 in]
        n114 = Negate(x=w230) -> (-x=w229:dbl)
      }
      frame "Arc Turn" {
        n115 = Add(x=w254, y=w253) -> (x+y=w261:dbl)
        n116 = call <vilib>:"Get_YPRHfH.vi"("Device Number"=FRIC_navX_DeviceNumbersTypeDef."Dev0") -> ("YRPHfH"=w257:T28)  [unwired: 10 in]
        n117 = Unbundle By Name(w257) -> ("Yaw"=w255:dbl)
        n118 = Subtract(x=w255, y=w261) -> (x-y=w263:dbl)
        n119 = Add(x=w263, y=180.0) -> (x+y=w266:dbl)
        n120 = Quotient & Remainder(x=w266, y=360.0) -> (x-y*floor(x/y)=w264:dbl)  [unwired: 1 out]
        n121 = Subtract(x=w264, y=180.0) -> (x-y=w260:dbl)
        n122 = In Range and Coerce(upper limit=1.0, x=w260, lower limit=-1.0) -> ()  [unwired: 2 out]
        n123 = call-poly <vilib>:"PID.vi"("output range"=cluster{"output high":dbl, "output low":dbl} {"output high"=0.5, "output low"=-0.5}, "PID gains"=T1 {"proportional gain (Kc)"=0.02, "integral time (Ti, min)"=0.0, "derivative time (Td, min)"=0.0}, "process variable"=w260, "setpoint"=0.0) -> ("output"=w251:dbl)  [unwired: 6 in, 1 out]
      }
      frame "Drive Path" {
        n124 = disable-structure shown="Enabled" {
          disable-tunnel: [w288 30.0 ("Trackwidth")] -> w273
          frame Disabled {
            n125 = global read "Constants.vi" "Track Width"() -> (w288:dbl)
          }
          frame Enabled {
          }
        }
        n126 = Unbundle(T30 {"dx/dt"=0.0, "dx/dt"=0.0, "Yaw"=0.0, {0.0, 0.0}} ("cluster")) -> ("dx/dt"=w280:dbl, "dx/dt"=w279:dbl, "Yaw"=w278:dbl, w277:cluster{dbl, dbl})
        n127 = Unbundle(w283) -> ("Iterations"=w274:i32)  [unwired: 1 out]
        n128 = Equal To 0?(x=w274) -> (x = 0?=w275:bool)
        n129 = Bundle(cluster=T31 {"LeftDistance"=0.0, "RightDistance"=0.0, "LeftVelocity"=0.0, "RightVelocity"=0.0, "Angle"=0.0, "Location"={0.0, 0.0}} ("SensorData"), "LeftVelocity"=w280, "RightVelocity"=w279, "Angle"=w278, "Location"=w277) -> (w281:T31)  [unwired: 2 in]
        n130 = call "PurePursuit.vi"("RobotNeededPathData"=w287, "SensorData"=w281, "Trackwidth"=w273, "Reset"=w275, "Gains"="Gains") -> ("LeftValue"=w286:dbl, "RightValue"=w285:dbl, "Done"=w284:bool)  [unwired: 6 in, 2 out]
      }
    }
    n131 = call "Drive Check for New Command.vi"("input cluster"=w95, "Wait time (ms)"=w121, "Finished?"=w120) -> ("Completion"=w123:T6, "Subsystem Name"=w117:string, "Current Command"=w118:T3, "Initial Trace String"=w119:string, "Next Command"=w122:T32)  [unwired: 4 in]
    n132 = Bundle("LeftValue"=w99, "RightValue"=w98) -> (→"Setpoints":cluster{"LeftValue":dbl, "RightValue":dbl})  [unwired: 1 in]
    n133 = global write "Drive Published Globals.vi" "MotorRight"(w98) -> ()
    n134 = global write "Drive Published Globals.vi" "MotorLeft"(w99) -> ()
    n135 = case shown="\"Successful\", \"Aborted\"" w123 {
      selector: w123 -> [_ w298]
      tunnel: w119 -> [_ w293]
      tunnel: w118 -> [_ w294]
      tunnel: w117 -> [_ w290]
      frame "Incomplete", Default {
        # "Continuing current command"
      }
      frame "Successful", "Aborted" {
        # "Report and setup for next command"
        n136 = Unbundle By Name(w294) -> ("Left Speed"=w296:dbl, "Right Speed"=w297:dbl, "Duration"=w291:dbl)
        n137 = Format Into String(format string="L %.1f, R %.1f, D %f", initial string=w293, w296, w297, w291) -> (resulting string=w292:string)  [unwired: 1 in, 1 out]
        "Current\nCmd" <- w292
        n138 = call <vilib>:"Trace Results.vi"("Status of previous command"=w298, "Description"=w292, "Subsystem"=w290) -> ()  [unwired: 9 in]
      }
    }
    n139 = call <vilib>:"WPI_RobotDriveMotors.vi"("RightSpeed"=w98, "LeftSpeed"=w99, "RobotDriveDevRef"=w104) -> ()  [unwired: 1 in, 8 out]
    n140 = call <vilib>:"WPI_RobotDriveMotors.vi"("RightSpeed"=w98, "LeftSpeed"=w99, "RobotDriveDevRef"=w103) -> ()  [unwired: 1 in, 8 out]
  }
